vi "Server.vi"() -> ()   [LabVIEW 2020]
uses:
  <vilib>/NI/Actors/Network Endpoint Actors/Protocols/TCP Strategy/TCP Stream Listener/TCP Stream Listener.lvclass
  C:/Program Files (x86)/National Instruments/LabVIEW 2020/vi.lib/NI/Actors/Network Endpoint Actors/Protocols/TCP Strategy/TCP Stream/TCP Stream.lvclass
  G:/Utilisateurs/hugofroylan.aragon/Documents/LabVIEW-Projects/Nested Endpoint Actors Optimized/Abstract Classes/Message Stream/Message Stream.lvclass
  Chat Window/Chat Window.lvclass
  C:/Program Files (x86)/National Instruments/LabVIEW 2020/vi.lib/ActorFramework/Actor/Actor.lvclass
  Nested Endpoint Actors/Serializer/Serializable Flattener/Serializable Flattener.lvclass
  G:/Utilisateurs/hugofroylan.aragon/Documents/LabVIEW-Projects/Nested Endpoint Actors Optimized/Abstract Classes/Message Flattener/Message Flattener.lvclass
  <vilib>/NI/Actors/Network Endpoint Actors/Protocols/TCP Strategy/TCP Stream/TCP Stream.lvclass/TCP Stream.ctl
  Chat Window Messages/Display Text Msg/Display Text Msg.lvclass
  Chat Window Messages/echo Msg/echo Msg.lvclass
  Chat Window Messages/echo reply Msg/echo reply Msg.lvclass
  Chat Window Messages/Update Number Msg/Update Number Msg.lvclass
  Chat Window/Chat Window.lvclass/Chat Window.ctl
  <vilib>/NI/Actors/Network Endpoint Actors/Protocols/TCP Strategy/TCP Stream/TCP Stream.lvclass
  <vilib>/ActorFramework/Actor/Actor.lvclass
panel:
  out "error out":errorcluster
  in  "local port":u16=2001
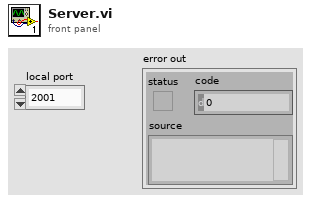
[diagram p1: front panel]
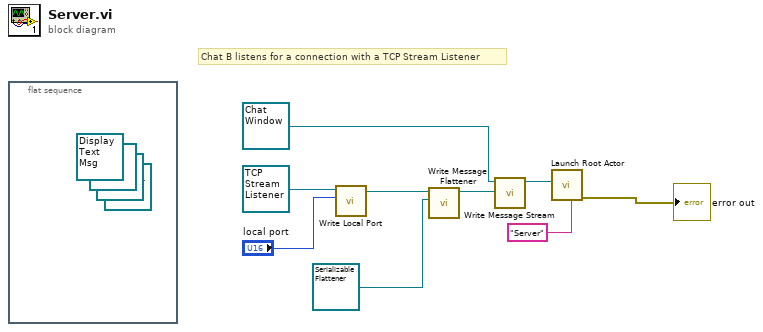
[diagram p0: block diagram]
diagram:
  # "Chat B listens for a connection with a TCP Stream Listener"
  n1 = flat-sequence {
    frame #0 {
      (unwired) refnum<class "Update Number Msg.lvclass"> refnum ("Chat Window.lvlib:Update Number Msg.lvclass")
      (unwired) refnum<class "echo reply Msg.lvclass"> refnum ("Chat Window.lvlib:echo reply Msg.lvclass")
      (unwired) refnum<class "echo Msg.lvclass"> refnum ("Chat Window.lvlib:echo Msg.lvclass")
      (unwired) refnum<class "Display Text Msg.lvclass"> refnum ("Chat Window.lvlib:Display Text Msg.lvclass")
    }
  }
  n2 = call <vilib>:"Write Local Port.vi"("local port"="local port", "TCP Stream in"=refnum<class "TCP Stream Listener.lvclass"> refnum ("TCP Stream Listener.lvclass")) -> ("TCP Stream out"=w3:refnum<class "TCP Stream Listener.lvclass">)  [unwired: 9 in]
  n3 = call-dynamic "Write Message Flattener.vi"("Message Flattener.lvclass"=refnum<class "Serializable Flattener.lvclass"> refnum ("Serializable Flattener Optimized.lvclass"), "Message Stream in"=w3) -> ("Message Stream out"=w2:refnum<class "TCP Stream Listener.lvclass">)  [unwired: 9 in]
  n4 = call "Write Message Stream.vi"("Message Stream"=w2, "Chat Window in"=refnum<class "Chat Window.lvclass"> refnum) -> ("Chat Window out"=w7:refnum<class "Chat Window.lvclass">)  [unwired: 9 in]
  n5 = call <vilib>:"Launch Root Actor.vi"("Debug Alias"="Server", "Actor"=w7) -> ("error out"=→"error out":errorcluster)  [unwired: 8 in, 1 out]
